vi "Attach Observer.vi"(10 "Observer(s)":refnum<class "Send.lvclass">, 11 "MGR.lvclass in":refnum<class "MGR.lvclass">) -> (3 "MGR.lvclass out":refnum<class "MGR.lvclass">)   [LabVIEW 2011, in "Messenging.lvlib" / "MGR.lvclass"]
uses:
  MGR.lvclass
  Send/Send.lvclass
  MGR.lvclass/MGR.ctl
  SendMultiple/ObserverSet.lvclass
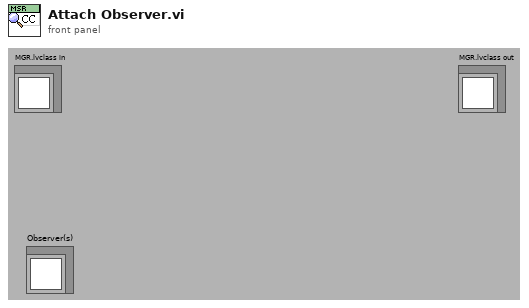
[diagram p1: front panel]
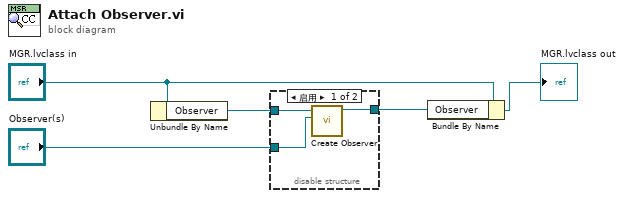
[diagram p0: block diagram]
diagram:
  n1 = Unbundle By Name("MGR.lvclass in") -> ("Observer"=w3:refnum<class "Observer.lvclass">)
  n2 = disable-structure shown="启用" {
    disable-tunnel: w3 -> [w8 _]
    disable-tunnel: "Observer(s)" -> [w7 w9]
    disable-tunnel: [w6 w9] -> w1
    frame Enabled {
      n3 = call "Create Observer.vi"("Additional Input"=w7, "Input"=w8) -> ("Observer"=w6:refnum<class "Observer.lvclass">)  [unwired: 7 out]
    }
    frame Disabled {
    }
  }
  n4 = Bundle By Name(cluster="MGR.lvclass in", "Observer"=w1) -> (→"MGR.lvclass out":refnum<class "MGR.lvclass">)
